vi "Main(Array).vi"() -> ()   [LabVIEW 2017]
doc: "The myRIO Project template acquires acceleration data from the onboard accelerometer and displays the changes of acceleration values in a waveform chart."
uses:
  <vilib>/Platform/TimedLoop/XDataNode/timing_clust.ctl
  <vilib>/Platform/TimedLoop/XDataNode/nitl_modes.ctl
  <vilib>/Platform/TimedLoop/XDataNode/wakeup.ctl
  <vilib>/FPGAPlugInAG/myRIO-1900/niLvFpga_Open_myRIO-1900.vi
  <vilib>/rvi/interface/common/dynamic/niFpgaDynamicAddResources.vi
  <vilib>/myRIO/Common/Instrument Driver Framework/Utilities/vis/FPGA Ref Manager.vi
  <vilib>/Utility/error.llb/Error Cluster From Error Code.vi
  <vilib>/myRIO/Common/Instrument Driver Framework/Utilities/vis/Ref Counter.vi
  <vilib>/rvi/errors/niLvFpgaAdjustHostInterfaceError.vi
  <vilib>/imath/engines/lvmath2/RunTimeEngine/NodeEndStatement/NIMS_NodeEndStatement_Output.vi
  <instcachedir>/0/NIMS_NodeEndStatement_Output_53EC0D466D134D7ABD903AC30B43404B.lvgen/NIMS_NodeEndStatement_Output_53EC0D466D134D7ABD903AC30B43404B_001.vi
  <vilib>/imath/engines/lvmath2/RunTimeEngine/ErrorHandling/NIMS_Finalize Error.vi
  <vilib>/FPGAPlugInAG/Dynamic/niLvFpga_Close_Dynamic.vi
  <vilib>/rvi/interface/nirviOpenFPGA/nirviOpenFPGA.xnode
  FPGA Bitfiles/FPGADEMO_FPGATarget_FPGAENCODER_OUiAhW3lqQo.lvbitx
  FPGA ENCODER.vi
  <vilib>/platform/TimedLoop/XDataNode/XDataNode.xnode
  <vilib>/rvi/interface/nirviReadWriteControl/nirviReadWriteControl.xnode
  <vilib>/rvi/interface/nirviCloseFPGA/nirviCloseFPGA.xnode
  <vilib>/Platform/TimedLoop/XDataNode/XDNodeRunTimeDep.lvlib
  <vilib>/myRIO/Instrument Drivers/Utilities/Utilities.lvlib
  NiFpgaLv.dll
  <vilib>/rvi/interface/Simulation/niFpgaSimulationCallBeginRW.vi
panel:
  in  "Freq":dbl
  out "Waveform Graph":dbl[][](graph)
  in  "Filter Counts":u16
  in  "Clear Overflow?":bool
  in  "Clear Error?":bool
  in  "Reset":bool
  in  "Pause?":bool
  in  "Clear Sigam?":bool
  in  "Reference Input":T1={"Amp"=0.0, "Fred"=0.01, "Offset"=0.0, "Type"=0.0} {"Offset" step=0.1; "Fred" min=0.001 step=0.1; "Amp" step=0.1}
  in  "PID Parameters":cluster{"Kp":dbl, "Ki":dbl, "Kd":dbl} {"Kd" step=0.1; "Ki" step=0.1; "Kp" step=0.1}
  out "Waveform Chart":T2(graph)
  in  "stop":bool
  out "error out":errorcluster
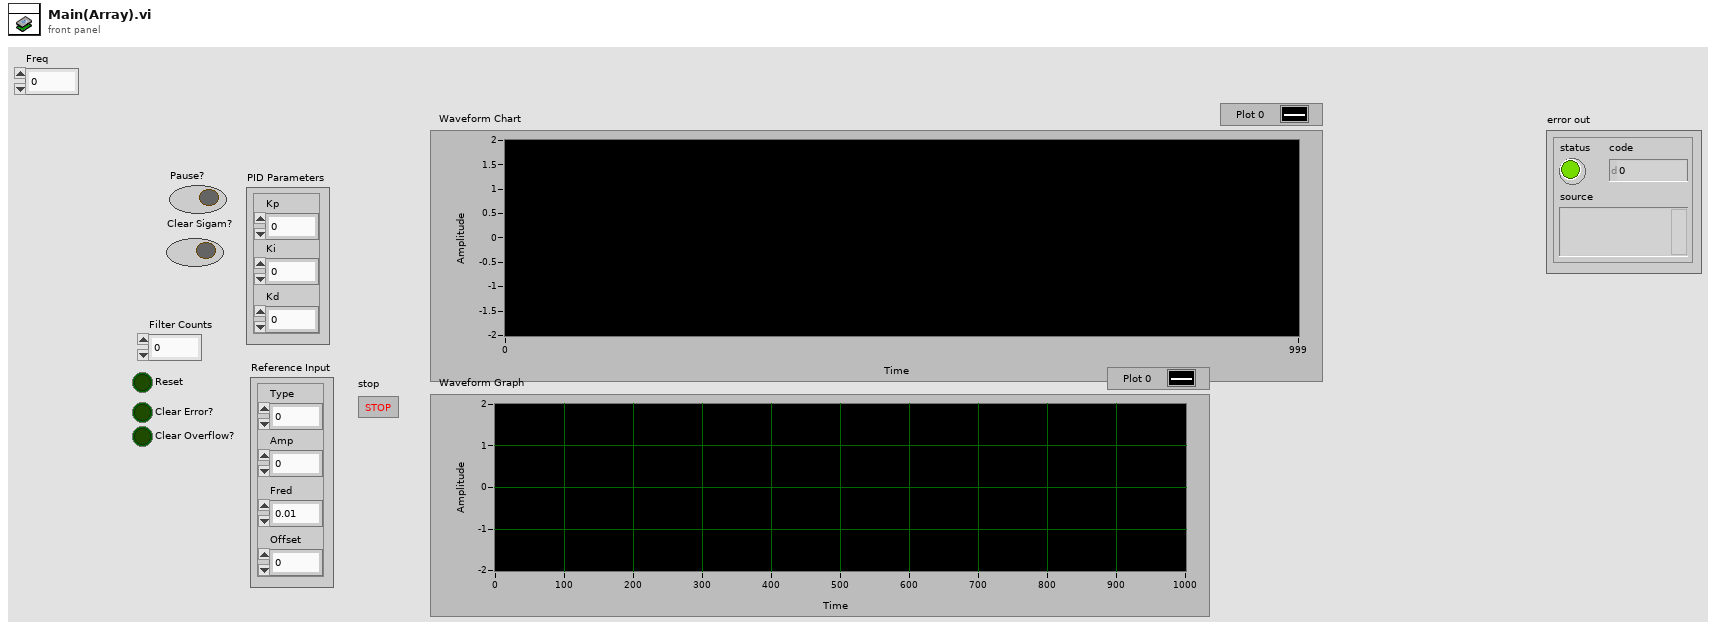
[diagram p1: front panel]
types:
  T1 = cluster{"Amp":dbl, "Fred":dbl, "Offset":dbl, "Type":dbl}
  T2 = cluster{"Output":dbl, dbl, "dbl Scaled Value":dbl}[]
  T3 = typedef "XDNodeRunTimeDep.lvlib/timing_clust.ctl" = cluster{"Expected End [f-1]":u64, "Actual End [f-1]":u64, "Finished Late? [f-1]":bool, "Expected End [i-1]":u64, "Actual End [i-1]":u64, "Finished Late? [i-1]":bool, "Expected Start [i]":u64, "Actual Start [i]":u64, "Expected Start [f]":u64, "Actual Start [f]":u64, "Source Name":string, "Structure Name":string, "Period":i64, "Deadline":i64, "Offset":i64, "Start":i64, "Priority":i32, "Timeout":i32, "Mode":T4, "Wakeup Reason":T5, "Error":errorcluster, "Source Type":string, "Secondary Source Type":string, "Global End Time":u64, "Global Start Time":u64, "Frame Duration":u64, "Iteration Duration":u64, "Assigned CPU":i32, "I/O Scan Engine Mode":u32}
  T4 = typedef "XDNodeRunTimeDep.lvlib/nitl_modes.ctl" = enum32{"No Change", "Process missed periods, maintain original phase", "Discard missed periods, maintain original phase", "Process missed periods, ignore original phase", "Discard missed periods, ignore original phase"}
  T5 = typedef "XDNodeRunTimeDep.lvlib/wakeup.ctl" = enum32{"Normal", "Aborted", "Asynchronous wakeup", "Timing source error", "Timed loop error", "Timeout"}
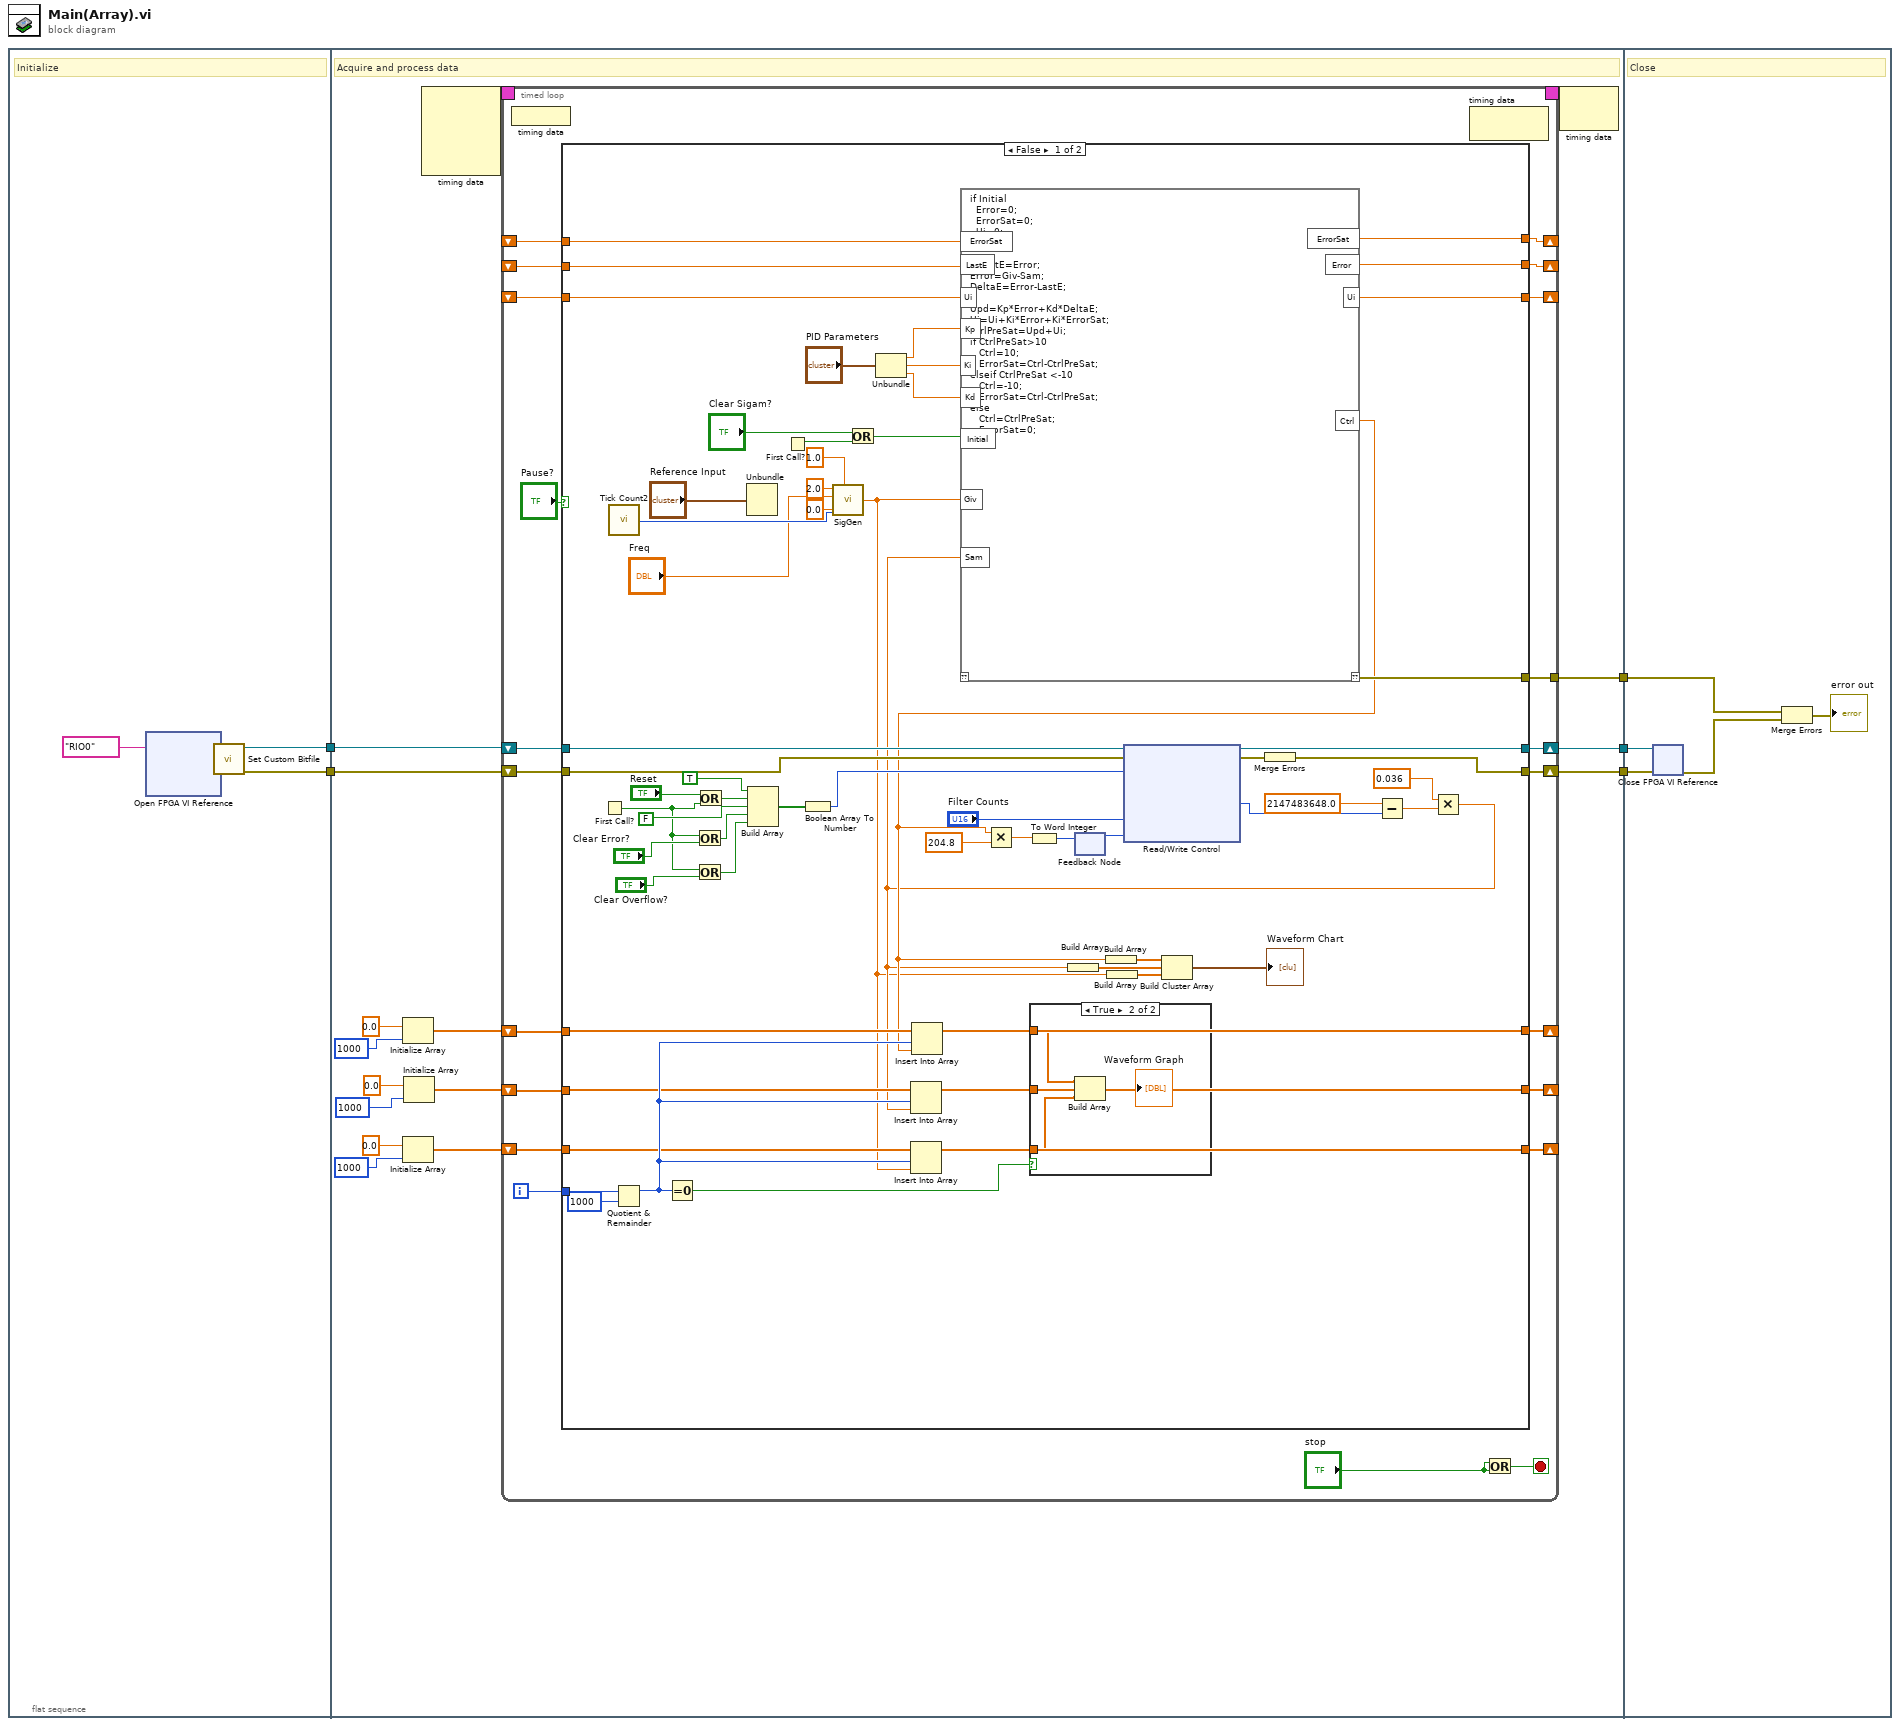
[diagram p0: block diagram]
diagram:
  n1 = flat-sequence {
    tunnel: [w7] -> w5
    tunnel: [w6] -> w4
    tunnel: w5 -> [w24]
    tunnel: w4 -> [w23]
    tunnel: [w22] -> w3
    tunnel: [w21] -> w2
    tunnel: [w20] -> w1
    tunnel: w3 -> [w300]
    tunnel: w2 -> [w299]
    tunnel: w1 -> [w297]
    frame #0 {
      # "Initialize"
      n2 = xnode "Open FPGA VI Reference"("resource name"=tag "RIO0") -> ("FPGA VI Reference Out"=w8:refnum<k20>, "error out"=w9:errorcluster)  [unwired: 1 in]
      n3 = call <vilib>:"Set Custom Bitfile.vi"("error in (no error)"=w9, "Custom FPGA Reference In"=w8) -> ("error out"=w6:errorcluster, "Custom FPGA Reference Out"=w7:refnum<k20>)  [unwired: 8 in]
    }
    frame #1 {
      # "Acquire and process data"
      n4 = Initialize Array(0.0 ("element"), 1000 ("dimension size")) -> (w11:dbl[])
      n5 = Initialize Array(0.0 ("element"), 1000 ("dimension size")) -> (w13:dbl[])
      n6 = Initialize Array(0.0 ("element"), 1000 ("dimension size")) -> (w12:dbl[])
      n7 = node-c288() -> (w26:T3)  [unwired: 4 in]
      n8 = timed-loop {
        timing: w26 -> [_]
        timing-out: [_] -> w25
        shift-right: [w42] -> _
        shift-left: _ -> [w47]
        shift-right: [w46] -> _
        shift-left: _ -> [w45]
        shift-right: [w44] -> _
        shift-left: _ -> [w43]
        shift-right: [w35] -> w22
        shift-left: w24 -> [w38]
        shift-right: [w36] -> w21
        shift-left: w23 -> [w37]
        tunnel: [w34] -> w20
        shift-right: [w32] -> _
        shift-left: w13 -> [w31]
        shift-right: [w29] -> _
        shift-left: w12 -> [w30]
        shift-right: [w27] -> _
        shift-left: w11 -> [w28]
        i -> [w33]
        stop <- w41 stop-if-true
        n9 = node-c288() -> ()  [unwired: 1 in]
        n10 = case shown="False" "Pause?" {
          tunnel: w47 -> [w105 w290]
          tunnel: [w104 w291] -> w46
          tunnel: w45 -> [w103 w291]
          tunnel: [w102 w292] -> w44
          tunnel: w43 -> [w101 w292]
          tunnel: [w97 w290] -> w42
          tunnel: w38 -> [w93 w289]
          tunnel: w37 -> [w92 w288]
          tunnel: [w75 w288] -> w36
          tunnel: [w74 w289] -> w35
          tunnel: [w73 _] -> w34
          tunnel: w33 -> [w72 _]
          tunnel: [w67 w287] -> w32
          tunnel: w31 -> [w66 w287]
          tunnel: w30 -> [w65 w285]
          tunnel: [w64 w285] -> w29
          tunnel: w28 -> [w63 w286]
          tunnel: [w62 w286] -> w27
          frame False {
            n11 = First Call?() -> (First Call?: T/F=w85:bool)
            n12 = call "Tick Count2"() -> ("Tick Count(uSec)"=w94:u32)
            n13 = Quotient & Remainder(x=w72, y=1000) -> (x-y*floor(x/y)=w69:i32)  [unwired: 1 out]
            n14 = Equal To 0?(x=w69) -> (x = 0?=w70:bool)
            n15 = Or(x=w85, y="Clear Error?") -> (x .or. y?=w84:bool)
            n16 = Or(x=w85, y="Clear Overflow?") -> (x .or. y?=w83:bool)
            n17 = Or(x="Reset", y=w85) -> (x .or. y?=w90:bool)
            n18 = Unbundle("Reference Input") -> ()  [unwired: 4 out]
            n19 = Build Array(TRUE, w90, FALSE, w84, w83) -> (w82:bool[])
            n20 = First Call?() -> (First Call?: T/F=w98:bool)
            n21 = Boolean Array To Number(Boolean array=w82) -> (number=w81:u32)
            n22 = call "SigGen.vi"("Amp"=2.0, "Freq"="Freq", "Offset"=0.0, "Timer"=w94, "Type"=1.0) -> ("Output"=w56:dbl)
            n23 = Or(x="Clear Sigam?", y=w98) -> (x .or. y?=w100:bool)
            n24 = Unbundle("PID Parameters") -> ("Kp"=w108:dbl, "Ki"=w107:dbl, "Kd"=w106:dbl)
            n25 = Insert Into Array(array=w66, index=w69, new element=w56) -> (w67:dbl[])
            n26 = feedback #1() -> (w54:i16)  [unwired: 1 in]
            n27 = Build Array(w56) -> (w68:dbl[])
            n28 = xnode "Read/Write Control"("FPGA VI Reference In"=w93, "error in"=w92, "CNFG"=w81, "Debounce Ticks"="Filter Counts", "ConnectorC/AO0"=w54) -> ("FPGA VI Reference Out"=w74:refnum<k20>, "error out"=w80:errorcluster, "CNTR"=w76:u32)  [unwired: 1 out]
            n29 = Merge Errors(w80) -> (w75:errorcluster)
            n30 = Subtract(x=2147483648.0, y=w76) -> (x-y=w78:dbl)
            n31 = Multiply(x=0.036, y=w78) -> (x*y=w57:dbl)
            n32 = Insert Into Array(array=w65, index=w69, new element=w57) -> (w64:dbl[])
            n33 = mathscript code="if Initial\n  Error=0;\n  ErrorSat=0;\n  Ui=0;\nend;\n\n%LastE=Error;\nError=Giv-Sam;\nDeltaE=Error-LastE;\n\nUpd=Kp*Error+Kd*DeltaE;\nUi=Ui+Ki*Error+Ki*ErrorSat;\nCtrlPreSat=Upd+Ui;\nif CtrlPreSat>10\n   Ctrl=10;\n   ErrorSat=Ctrl-CtrlPreSat;\nelseif CtrlPreSat <-10\n   Ctrl=-10;\n   ErrorSat=Ctrl-CtrlPreSat;\nelse \n   Ctrl=CtrlPreSat;\n   ErrorSat=0;\nend;"("Giv"=w56, "Sam"=w57, "Kp"=w108, "Ki"=w107, "Kd"=w106, "Ui"=w105, "Initial"=w100, "LastE"=w103, "ErrorSat"=w101) -> ("??"=w73:errorcluster, "Ctrl"=w61:dbl, "Ui"=w97:dbl, "Error"=w104:dbl, "ErrorSat"=w102:dbl)  [unwired: 1 in]
            n34 = Insert Into Array(array=w63, index=w69, new element=w61) -> (w62:dbl[])
            n35 = Multiply(x=w61, y=204.8) -> (x*y=w60:dbl)
            n36 = To Word Integer(number=w60) -> (16bit integer=w55:i16)
            n37 = case shown="True" w70 {
              tunnel: w62 -> [_ w111]
              tunnel: w64 -> [_ w112]
              tunnel: w67 -> [_ w110]
              frame False {
              }
              frame True {
                n38 = Build Array(w111, w112, w110) -> ()  [unwired: 1 out]
              }
            }
            n39 = Build Array(w57) -> (w95:dbl[])
            n40 = feedback-in #1(w55) -> ()
            n41 = Build Array(w61) -> (w96:dbl[])
            n42 = Build Cluster Array(w96, w95, w68) -> (→"Waveform Chart":cluster{"Ctrl":dbl, dbl, "Output":dbl}[])
          }
          frame True {
          }
        }
        n43 = node-c288() -> ()  [unwired: 1 in, 1 out]
        n44 = Or(x="stop", y="stop") -> (x .or. y?=w41:bool)
      }
      n45 = node-c288(w25) -> ()  [unwired: 1 out]
    }
    frame #2 {
      # "Close"
      n46 = xnode "Close FPGA VI Reference"("FPGA VI Reference In"=w300, "error in"=w299) -> ("error out"=w298:errorcluster)
      n47 = Merge Errors(w297, w298) -> (→"error out":errorcluster)
    }
  }
